vi "Translate Stamp Calibration 2.vi"() -> ()   [LabVIEW 2011]
uses:
  Shared Components/Config Manager Class/Type Definitions/Part Type.ctl
  Shared Components/Vec3d Class/Vec3d Class.lvclass
  Shared Components/Config Manager Class/Config Manager Class.lvclass
panel:
  out "net rotation":dbl
  out "brass piece rotation":dbl
  out "stamp offset":cluster{dbl, dbl, dbl}
  in  "stamp offset start":i32=1
  in  "Stamp Offset config":path
  out "HDI XYZ":T1
  in  "Config Files Directory":path
  out "Stamp XYZ":T2
  in  "stamp start number":i32=1
  in  "PCA Config File":path
  out "Orient3d String":string
  out "Vec3d String":string
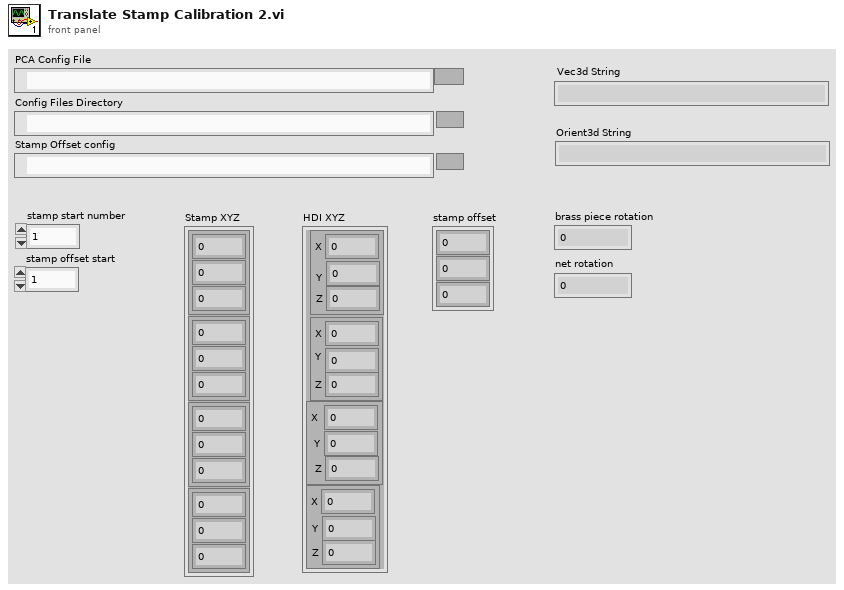
[diagram p1: front panel]
types:
  T1 = cluster{cluster{"X":dbl, "Y":dbl, "Z":dbl}, cluster{"X":dbl, "Y":dbl, "Z":dbl}, cluster{"X":dbl, "Y":dbl, "Z":dbl}, cluster{"X":dbl, "Y":dbl, "Z":dbl}}
  T2 = cluster{cluster{dbl, dbl, dbl}, cluster{dbl, dbl, dbl}, cluster{dbl, dbl, dbl}, cluster{dbl, dbl, dbl}}
  T3 = typedef "Part Type.ctl" = enum16{"BBM", "HDI", "BARE HDI", "GLUERESERVOIR", "STAMP_1", "STAMP_2", "STAMP_3", "STAMP_4", "STAMP_5", "WEIGHT_1", "WEIGHT_2", "WEIGHT_3", "WEIGHT_4", "WEIGHT_5", "WEIGHT_6", "WEIGHT_7", "WEIGHT_8", "PICKER_TOOL", "GRABER_TOOL"}
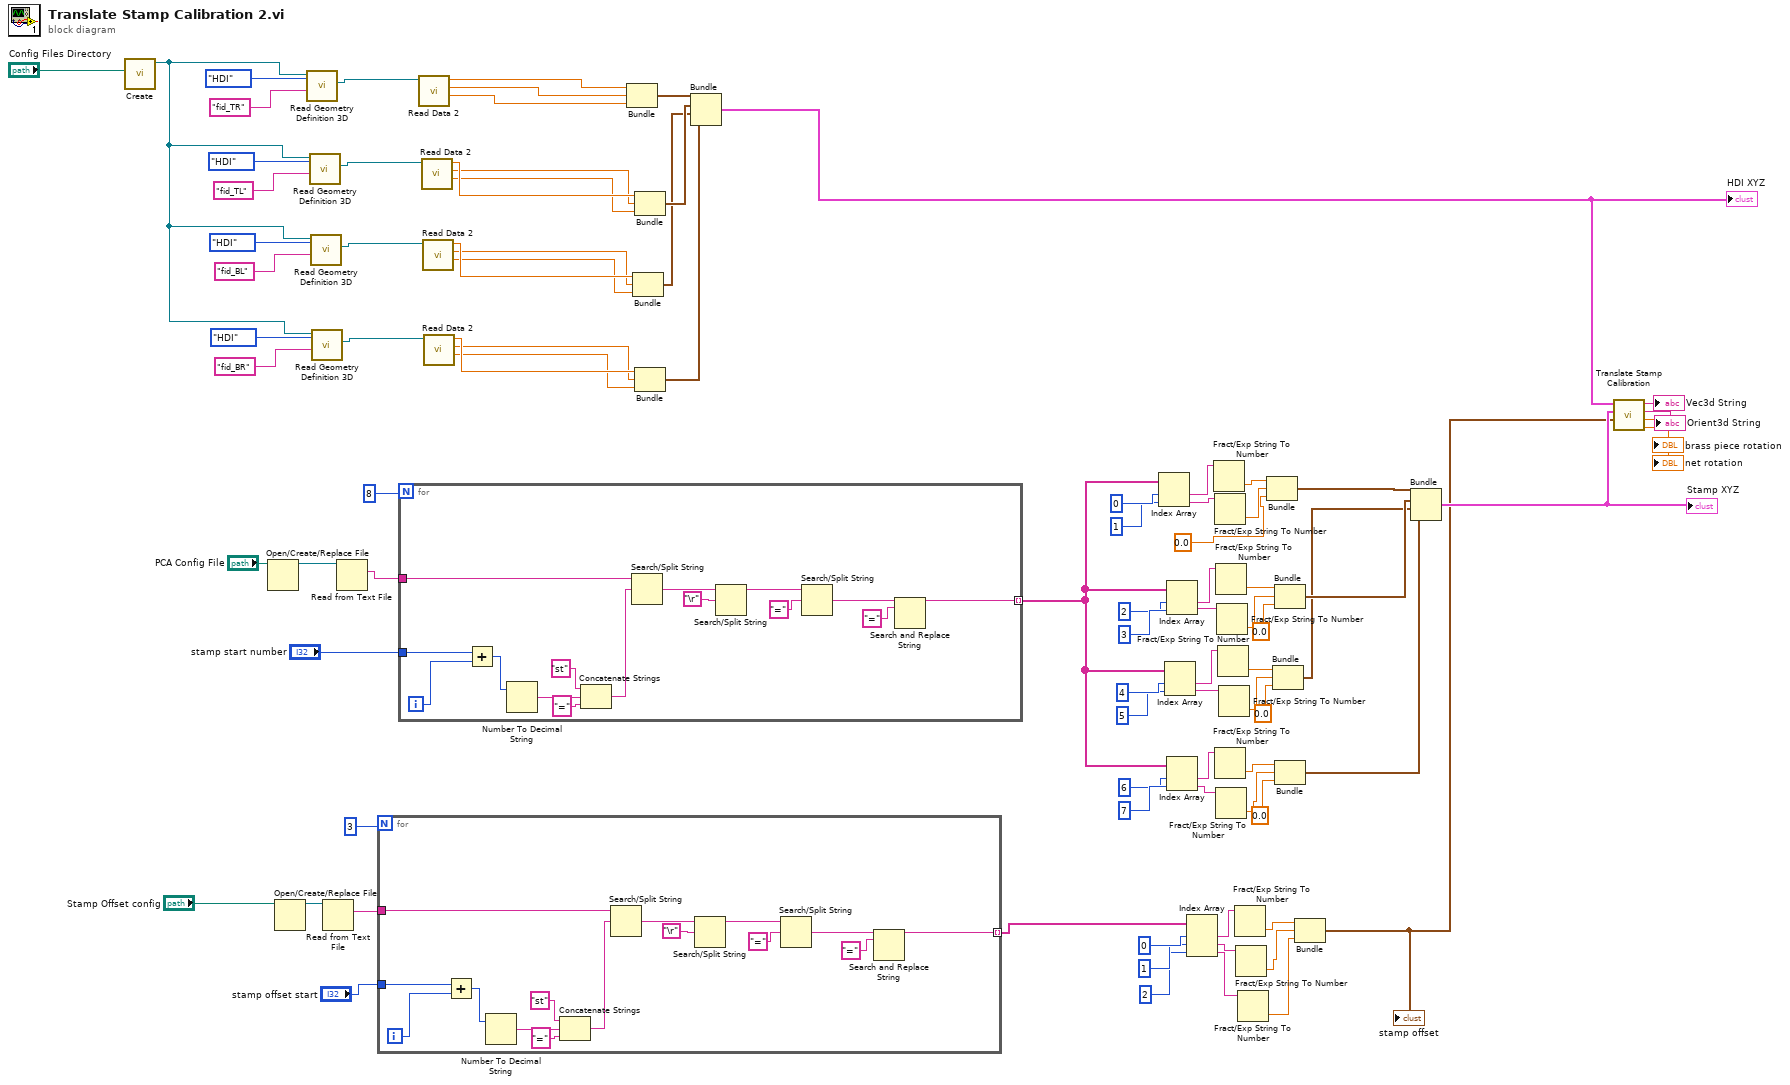
[diagram p0: block diagram]
diagram:
  n1 = call "Create.vi"("Config Files Directory"="Config Files Directory") -> ("Config Manager out"=w33:refnum<class "Config Manager Class.lvclass">)  [unwired: 9 in, 1 out]
  n2 = Open/Create/Replace File(file path (use dialog)="PCA Config File") -> (refnum out=w86:refnum<file>)  [unwired: 5 in, 2 out]
  n3 = Open/Create/Replace File(file path (use dialog)="Stamp Offset config") -> (refnum out=w18:refnum<file>)  [unwired: 5 in, 2 out]
  n4 = call "Read Geometry Definition 3D.vi"("Feature"="fid_TR", "Part Type"=Part_Type."HDI", "Config Manager in"=w33) -> ("Feature Coordinates"=w46:refnum<class "Vec3d Class.lvclass">)  [unwired: 6 in, 2 out]
  n5 = call "Read Geometry Definition 3D.vi"("Feature"="fid_TL", "Part Type"=Part_Type."HDI", "Config Manager in"=w33) -> ("Feature Coordinates"=w42:refnum<class "Vec3d Class.lvclass">)  [unwired: 6 in, 2 out]
  n6 = call "Read Geometry Definition 3D.vi"("Feature"="fid_BL", "Part Type"=Part_Type."HDI", "Config Manager in"=w33) -> ("Feature Coordinates"=w37:refnum<class "Vec3d Class.lvclass">)  [unwired: 6 in, 2 out]
  n7 = call "Read Geometry Definition 3D.vi"("Feature"="fid_BR", "Part Type"=Part_Type."HDI", "Config Manager in"=w33) -> ("Feature Coordinates"=w36:refnum<class "Vec3d Class.lvclass">)  [unwired: 6 in, 2 out]
  n8 = Read from Text File(file (use dialog)=w18) -> (text=w16:string)  [unwired: 3 in, 3 out]
  n9 = Read from Text File(file (use dialog)=w86) -> (text=w85:string)  [unwired: 3 in, 3 out]
  n10 = for {
    N: 3 -> [_]
    tunnel: w16 -> [w95]
    tunnel: "stamp offset start" -> [w94]
    tunnel: [w91] -> w7 mode=indexing
    i -> [w93]
    n11 = Add(x=w94, y=w93) -> (x+y=w92:i32)
    n12 = Number To Decimal String(number=w92) -> (decimal integer string=w103:string)  [unwired: 1 in]
    n13 = Concatenate Strings("st" ("string"), w103, "=" ("string")) -> (w105:string)
    n14 = Search/Split String(string=w95, search string/char (-)=w105) -> (match + rest of string=w96:string)  [unwired: 1 in, 2 out]
    n15 = Search/Split String(string=w96, search string/char (-)="\r") -> (substring before match=w99:string)  [unwired: 1 in, 2 out]
    n16 = Search/Split String(string=w99, search string/char (-)="=") -> (match + rest of string=w100:string)  [unwired: 1 in, 2 out]
    n17 = Search and Replace String(input string=w100, search string="=") -> (result string=w91:string)  [unwired: 6 in, 3 out]
  }
  n18 = for {
    N: 8 -> [_]
    tunnel: w85 -> [w110]
    tunnel: "stamp start number" -> [w109]
    tunnel: [w106] -> w75 mode=indexing
    i -> [w108]
    n19 = Add(x=w109, y=w108) -> (x+y=w107:i32)
    n20 = Number To Decimal String(number=w107) -> (decimal integer string=w118:string)  [unwired: 1 in]
    n21 = Concatenate Strings("st" ("string"), w118, "=" ("string")) -> (w120:string)
    n22 = Search/Split String(string=w110, search string/char (-)=w120) -> (match + rest of string=w111:string)  [unwired: 1 in, 2 out]
    n23 = Search/Split String(string=w111, search string/char (-)="\r") -> (substring before match=w114:string)  [unwired: 1 in, 2 out]
    n24 = Search/Split String(string=w114, search string/char (-)="=") -> (match + rest of string=w115:string)  [unwired: 1 in, 2 out]
    n25 = Search and Replace String(input string=w115, search string="=") -> (result string=w106:string)  [unwired: 6 in, 3 out]
  }
  n26 = call-dynamic "Read Data 2.vi"("Vec3d in"=w46) -> ("Z"=w29:dbl, "Y"=w44:dbl, "X"=w45:dbl)  [unwired: 7 in, 1 out]
  n27 = call-dynamic "Read Data 2.vi"("Vec3d in"=w42) -> ("Z"=w30:dbl, "Y"=w31:dbl, "X"=w32:dbl)  [unwired: 7 in, 1 out]
  n28 = call-dynamic "Read Data 2.vi"("Vec3d in"=w37) -> ("Z"=w26:dbl, "Y"=w27:dbl, "X"=w28:dbl)  [unwired: 7 in, 1 out]
  n29 = call-dynamic "Read Data 2.vi"("Vec3d in"=w36) -> ("Z"=w23:dbl, "Y"=w24:dbl, "X"=w25:dbl)  [unwired: 7 in, 1 out]
  n30 = Bundle("X"=w45, "Y"=w44, "Z"=w29) -> (w43:cluster{"X":dbl, "Y":dbl, "Z":dbl})  [unwired: 1 in]
  n31 = Bundle("X"=w28, "Y"=w27, "Z"=w26) -> (w21:cluster{"X":dbl, "Y":dbl, "Z":dbl})  [unwired: 1 in]
  n32 = Bundle("X"=w32, "Y"=w31, "Z"=w30) -> (w22:cluster{"X":dbl, "Y":dbl, "Z":dbl})  [unwired: 1 in]
  n33 = Bundle("X"=w25, "Y"=w24, "Z"=w23) -> (w20:cluster{"X":dbl, "Y":dbl, "Z":dbl})  [unwired: 1 in]
  n34 = Bundle(w43, w22, w21, w20) -> (w19:T1)  [unwired: 1 in]
  "HDI XYZ" <- w19
  n35 = Index Array(array=w75, index #1=0 ("index"), index #2=1 ("index")) -> (element #1=w69:string, element #2=w67:string)
  n36 = Index Array(array=w75, index #1=4 ("index"), index #2=5 ("index")) -> (element #1=w58:string, element #2=w59:string)
  n37 = Index Array(array=w75, index #1=2 ("index"), index #2=3 ("index")) -> (element #1=w61:string, element #2=w60:string)
  n38 = Index Array(array=w75, index #1=6 ("index"), index #2=7 ("index")) -> (element #1=w53:string, element #2=w54:string)
  n39 = Index Array(array=w7, index #1=0 ("index"), index #2=1 ("index"), index #3=2 ("index")) -> (element #1=w11:string, element #2=w10:string, element #3=w4:string)
  n40 = Fract/Exp String To Number(string=w69) -> (number=w68:dbl)  [unwired: 3 in, 1 out]
  n41 = Fract/Exp String To Number(string=w67) -> (number=w66:dbl)  [unwired: 3 in, 1 out]
  n42 = Fract/Exp String To Number(string=w53) -> (number=w52:dbl)  [unwired: 3 in, 1 out]
  n43 = Fract/Exp String To Number(string=w61) -> (number=w63:dbl)  [unwired: 3 in, 1 out]
  n44 = Fract/Exp String To Number(string=w54) -> (number=w50:dbl)  [unwired: 3 in, 1 out]
  n45 = Fract/Exp String To Number(string=w60) -> (number=w64:dbl)  [unwired: 3 in, 1 out]
  n46 = Fract/Exp String To Number(string=w58) -> (number=w57:dbl)  [unwired: 3 in, 1 out]
  n47 = Fract/Exp String To Number(string=w59) -> (number=w56:dbl)  [unwired: 3 in, 1 out]
  n48 = Fract/Exp String To Number(string=w11) -> (number=w12:dbl)  [unwired: 3 in, 1 out]
  n49 = Fract/Exp String To Number(string=w10) -> (number=w13:dbl)  [unwired: 3 in, 1 out]
  n50 = Fract/Exp String To Number(string=w4) -> (number=w3:dbl)  [unwired: 3 in, 1 out]
  n51 = Bundle(w68, w66, 0.0) -> (w70:cluster{dbl, dbl, dbl})  [unwired: 1 in]
  n52 = Bundle(w57, w56, 0.0) -> (w73:cluster{dbl, dbl, dbl})  [unwired: 1 in]
  n53 = Bundle(w63, w64, 0.0) -> (w74:cluster{dbl, dbl, dbl})  [unwired: 1 in]
  n54 = Bundle(w52, w50, 0.0) -> (w72:cluster{dbl, dbl, dbl})  [unwired: 1 in]
  n55 = Bundle(w12, w13, w3) -> (w5:cluster{dbl, dbl, dbl})  [unwired: 1 in]
  "stamp offset" <- w5
  n56 = Bundle(w70, w74, w73, w72) -> (w71:T2)  [unwired: 1 in]
  "Stamp XYZ" <- w71
  n57 = call "Translate Stamp Calibration.vi"("Known HDI Fiducials Coordinates"=w19, "Known Stamp Tool Coordinates"=w71, "Known Stamp Offsets"=w5) -> ("Vec3d String"=→"Vec3d String":string, "Orient3d String"=→"Orient3d String":string, "brass piece rotation"=→"brass piece rotation":dbl, "net rotation"=→"net rotation":dbl)  [unwired: 4 in]
